vi "CV.vi"(2 "Run uninterrupted?":bool, 3 "Device Category:":string(combo)="Short Strip", 4 "Batch No.:":string, 5 "Wafer Serial No.:":string, 6 "Sensor Serial No.:":string) -> (0 "Done!":bool)   [LabVIEW 2013]
doc: "Performs CV measurements according to ATLAS ITk Quality Control Specifications."
uses:
  InstrControl/Switching/Switching.lvclass
  InstrControl/SupplyControl/SupplyControl.lvclass
  InstrControl/LCRControl/LCRControl.lvclass
  general_VIs/globals/QC_MeasurementSetup.vi
  general_VIs/globals/QC_RunInformation.vi
  InstrControl/InstrumentSetup.vi
  InstrControl/ArduinoControl/ArduinoControl.lvclass
  <vilib>/Analysis/NI_AALBase.lvlib
  InstrControl/InstrControl.lvclass
panel:
  out "Frequency [Hz]":i32=1000 format="%#.3p"
  out "Resistance":dbl[](array[numeric]) caption="Res [kOhm]"
  out "Initial volts [V]":dbl format="%.1f"
  out "Final volts [V]":dbl=-700.0 format="%.1f"
  out "step [V]":dbl=10.0 format="%.1f"
  out "step interval [s]":u32=5
  out "Volts":dbl[](array[numeric]) caption="Volts [V]"
  out "Capacitance":dbl[](array[numeric]) caption="Cap [pF]"
  out "Temp.":dbl[](array[numeric]) caption="Temp. [°C]" format="%#.2f"
  out "RH":dbl[](array[numeric]) caption="RH [%]" format="%#.2f"
  out "Cgraph":cluster{"Initial volts":dbl, dbl, dbl[]}(graph)
  in  "Scales":T1(ring)
  in  "Cscale":enum16{"1/C^2 [1/nF^2]", "nF", "pF"}(ring)
  out "positive ramp?":bool
  out "Tab Control":enum32{"CV Setup", "CV Scan"}(tab)
  in  "Frequency [Hz] Setup":i32=1000 caption="Frequency [Hz]" format="%#.3p"
  in  "LCR Meter":string(combo)="WayneKerr 6440B"
  in  "User:":string(combo)="Christoph"
  in  "CV Supply":string(combo)="Keithley 2410"
  in  "Configurations":bool
  in  "Set\ncurrent\nlimit?":bool
  in  "Current \nLimit \n[µA]":dbl=1000.0 min=0.0001 format="%.3f"
  in  "Manufacturer:":string(combo)="Hamamatsu"
  in  "Quit":bool
  in  "Continue":bool
  in  "Temperature":enum16{"Read Arduino", "Enter manually"}(ring)
  in  "abort":bool
  out "Device Category:":string
  out "Batch:":string
  out "Current Volts:":dbl format="%.2f"
  in  "quit (no save)":bool
  in  "Quit & Save":bool
  out "Bias On/Off:":bool
  out "STATUS 1":string
  out "Initiated:":string
  out "Sensor No.:":string
  out "No of steps":u32
  out "Current reading No.":u32
  out "Last reading at:":string
  # "University of\nCambridge"
  # "Strip Sensor QC: CV"
  # "CV Scan parameters:"
  # "Last 5 readings:"
  # "n-4"
  # "n-3"
  # "n-2"
  # "n-1"
  # "n"
  # "Vertical Scale:"
  # "DUT & Test Description"
  # "Hardware"
  # "DUT & Test Description:"
  # "Current status:"
  # "Rdg No:"
  # "out of"
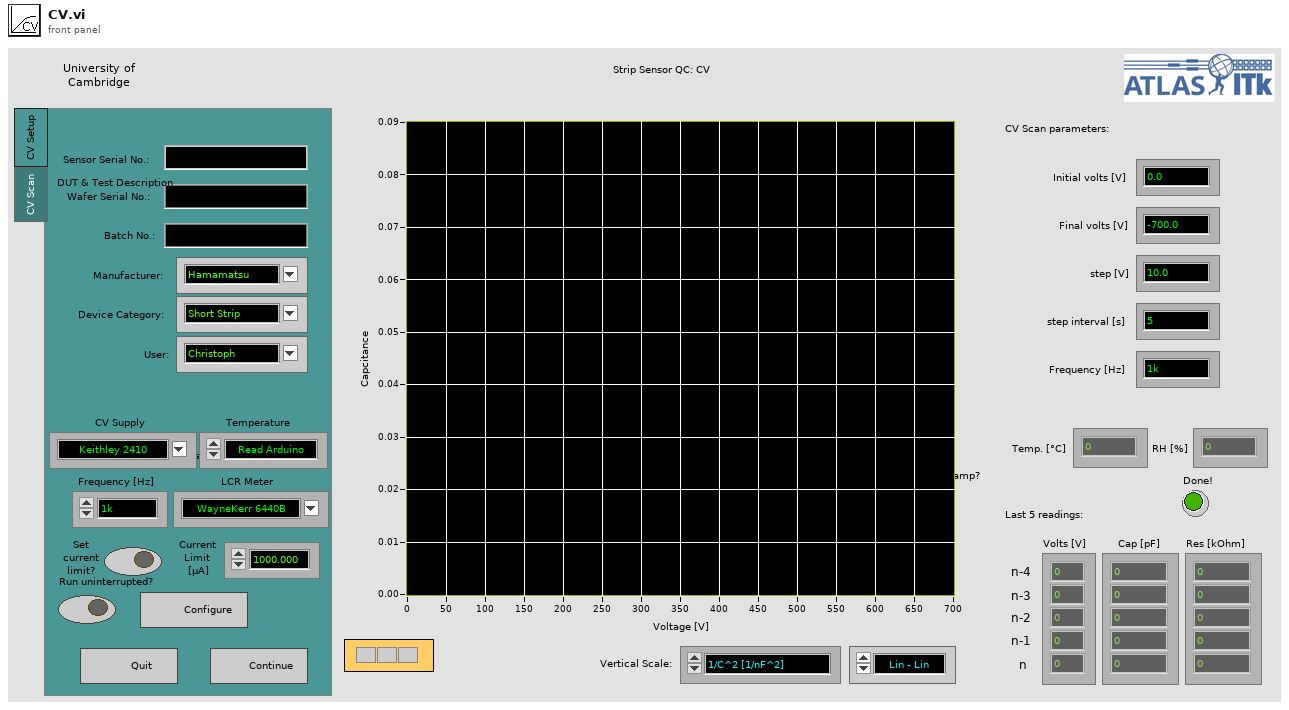
[diagram p1: front panel]
types:
  T1 = enum16{"Lin - Lin", "Log - Lin", "Lin - Log", "Log - log"}
  T2 = enum32{"IV", "CV", "Stability", "Striptest", "Cis", "Ris", "PTP"}
  T3 = enum16{"Reset", "Read Array", "Read Element", "Write Element", "Write Array", "Add Element", "Add Array"}
  T4 = enum16{"Reset", "Ground", "Striptest SMU", "Striptest LCR", "IV", "CV", "Interstrip Cap", "Interstrip Res"}
  T5 = cluster{"Sensor Serial No.:":string, "Wafer Serial No.:":string, "Batch:":string, "Manufacturer:":string, "Device Category:":string, "Database Serial No.:":string, "Initiated:":string, "Test":string, "Instruments used:":string, "Probeplan used:":string, "End of Run comment:":string, "User:":string}
  T6 = cluster{"Institute":string, "Manufacturers":string[], "Devices":string[], "Serialnumbers Lookup DB":string, "Data directory":string, "Backup & screenshot directory":string, "List of known users":string[]}
  T7 = cluster{"Supply":refnum<class "SupplyControl.lvclass">, "LCR":refnum<class "LCRControl.lvclass">, "Initial Voltage [V]":dbl, "Final Voltage [V]":dbl, "Step Size [V]":dbl, "Step Interval [s]":i32, "Number Of Steps":u32, "AC frequency [Hz]":i32, "RC Configuration":u16, "AC amplitude [V]":dbl, "Ramp down steps [V]":dbl, "Ramp down Interval [s]":i32, "Set Current Limit?":bool, "Current Limit [µA]":dbl, "Temperature Readout":enum16{"Read Arduino", "Enter manually"}, "Arduino":refnum<class "ArduinoControl.lvclass">, "Supply Name":string, "LCR Name":string, "V_depletion Limit [V]":dbl}
  T8 = cluster{"VISA address":refnum<visa-resource-name>, "T sensor":enum16{"SHT", "DS"}, "Arduino":refnum<class "ArduinoControl.lvclass">}
  T9 = cluster{"GPIB address":string, "Matrix address":string, "Mux1 address":string, "Mux2 address":string, "Matrix used?":bool, "Switching":refnum<class "Switching.lvclass">}
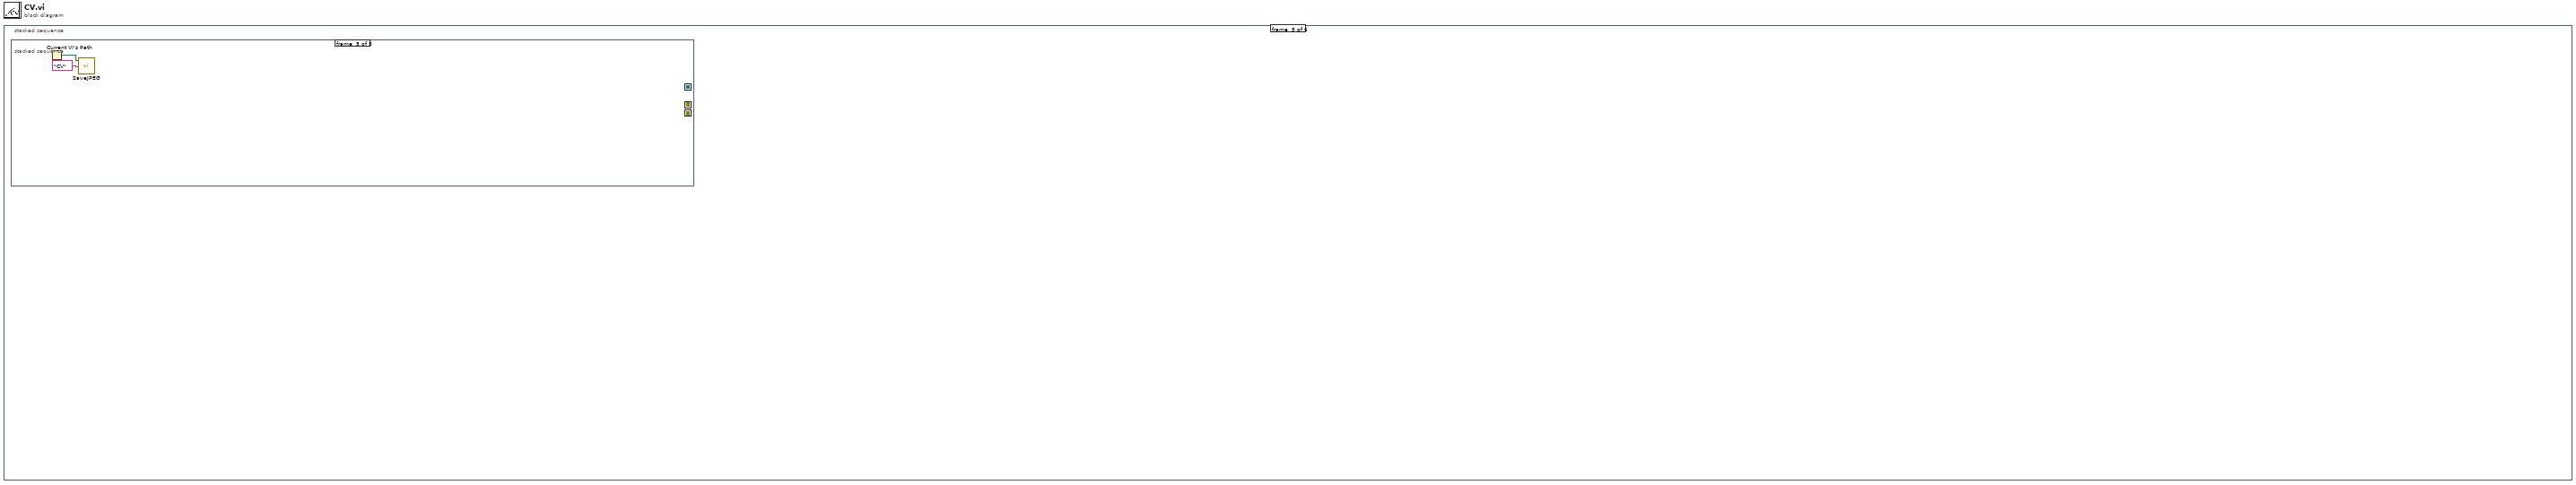
[diagram p0: block diagram]
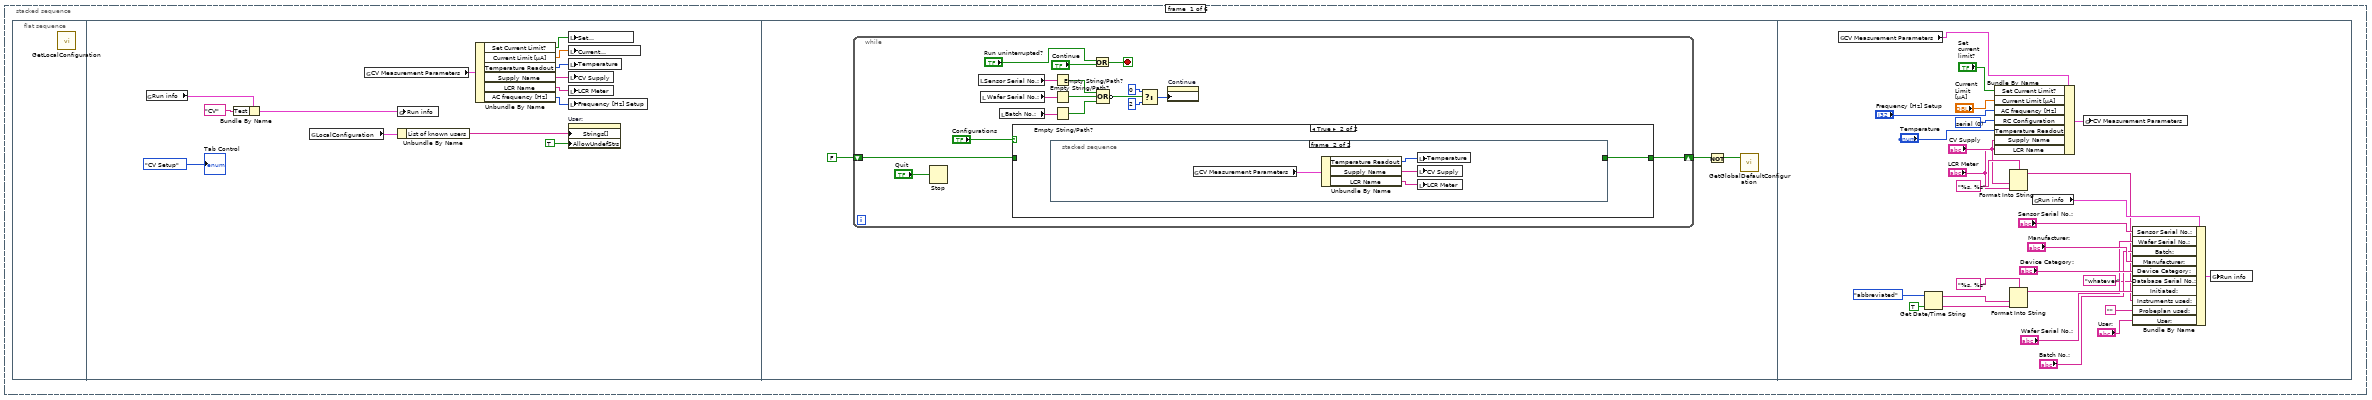
[diagram p2: hidden frame]
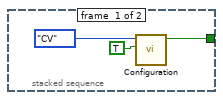
[diagram p4: hidden frame]
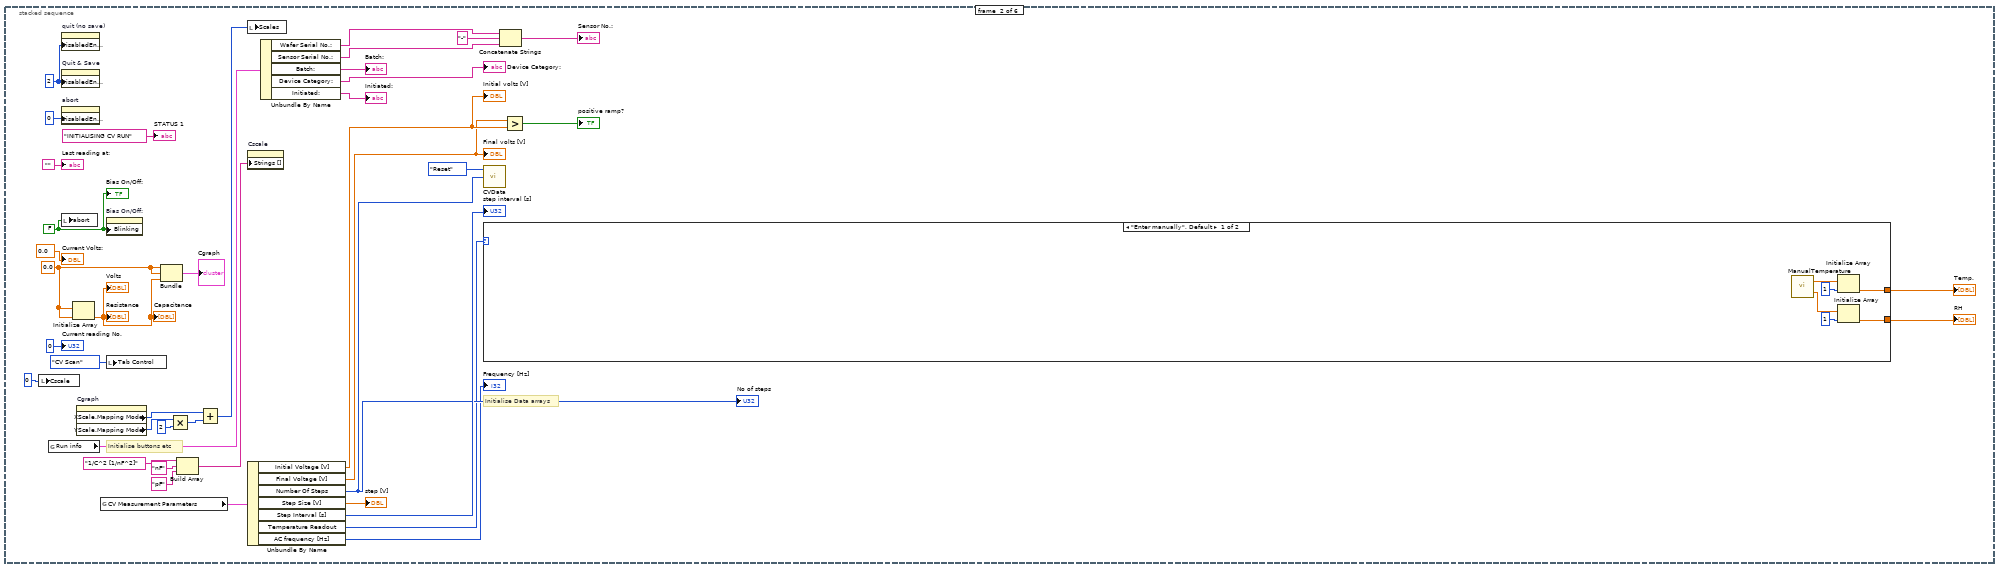
[diagram p5: hidden frame]
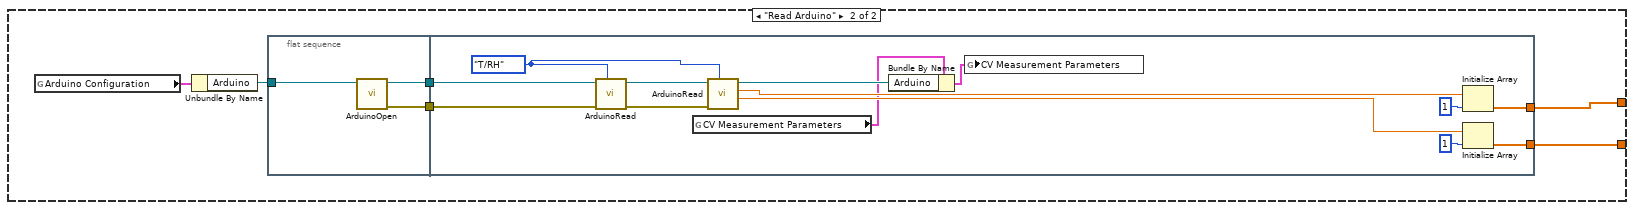
[diagram p6: hidden frame]
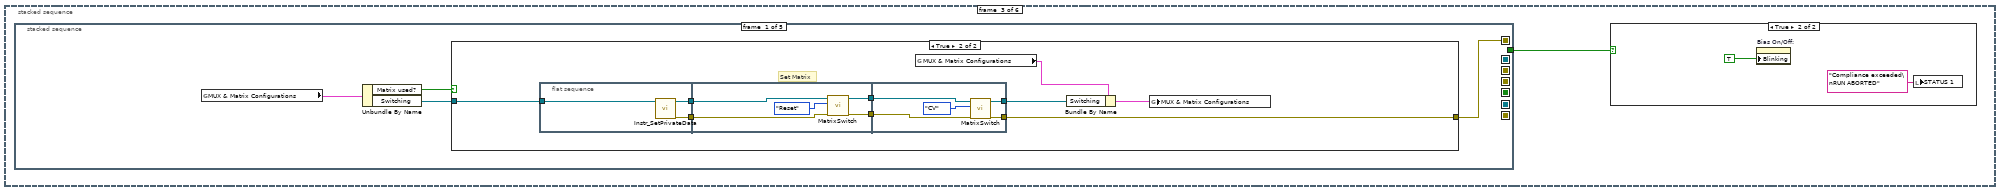
[diagram p7: hidden frame]
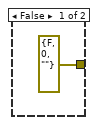
[diagram p8: hidden frame]
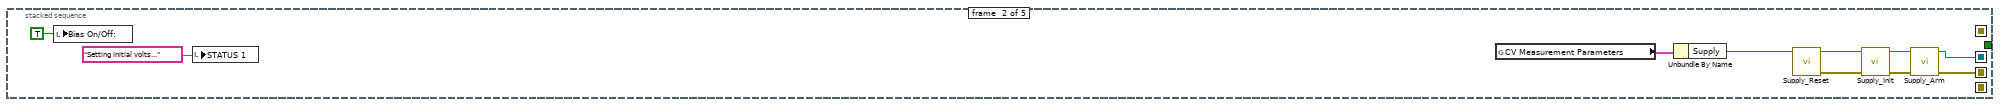
[diagram p9: hidden frame]
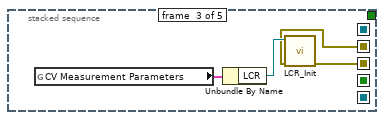
[diagram p10: hidden frame]
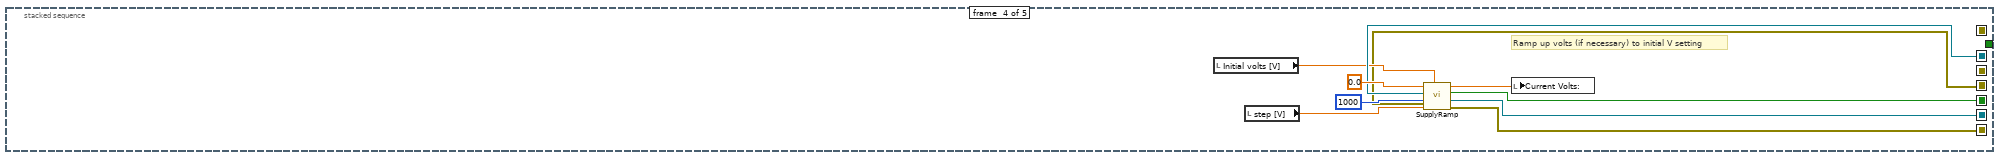
[diagram p11: hidden frame]
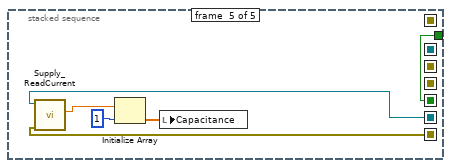
[diagram p12: hidden frame]
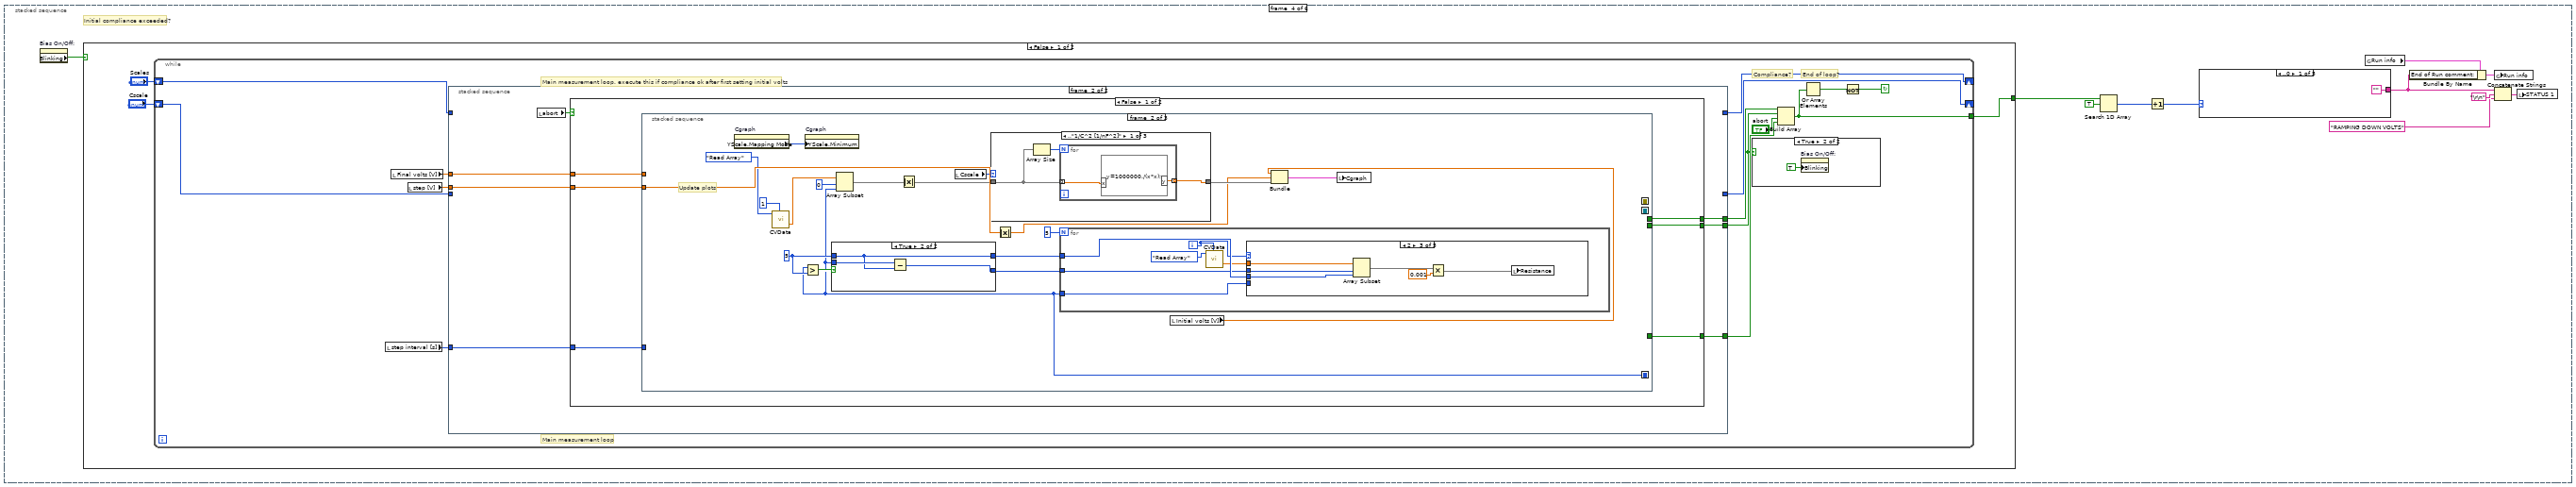
[diagram p14: hidden frame]
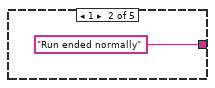
[diagram p15: hidden frame]
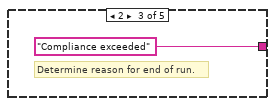
[diagram p16: hidden frame]
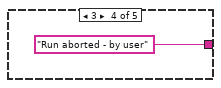
[diagram p17: hidden frame]
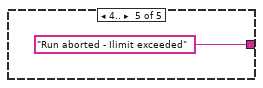
[diagram p18: hidden frame]
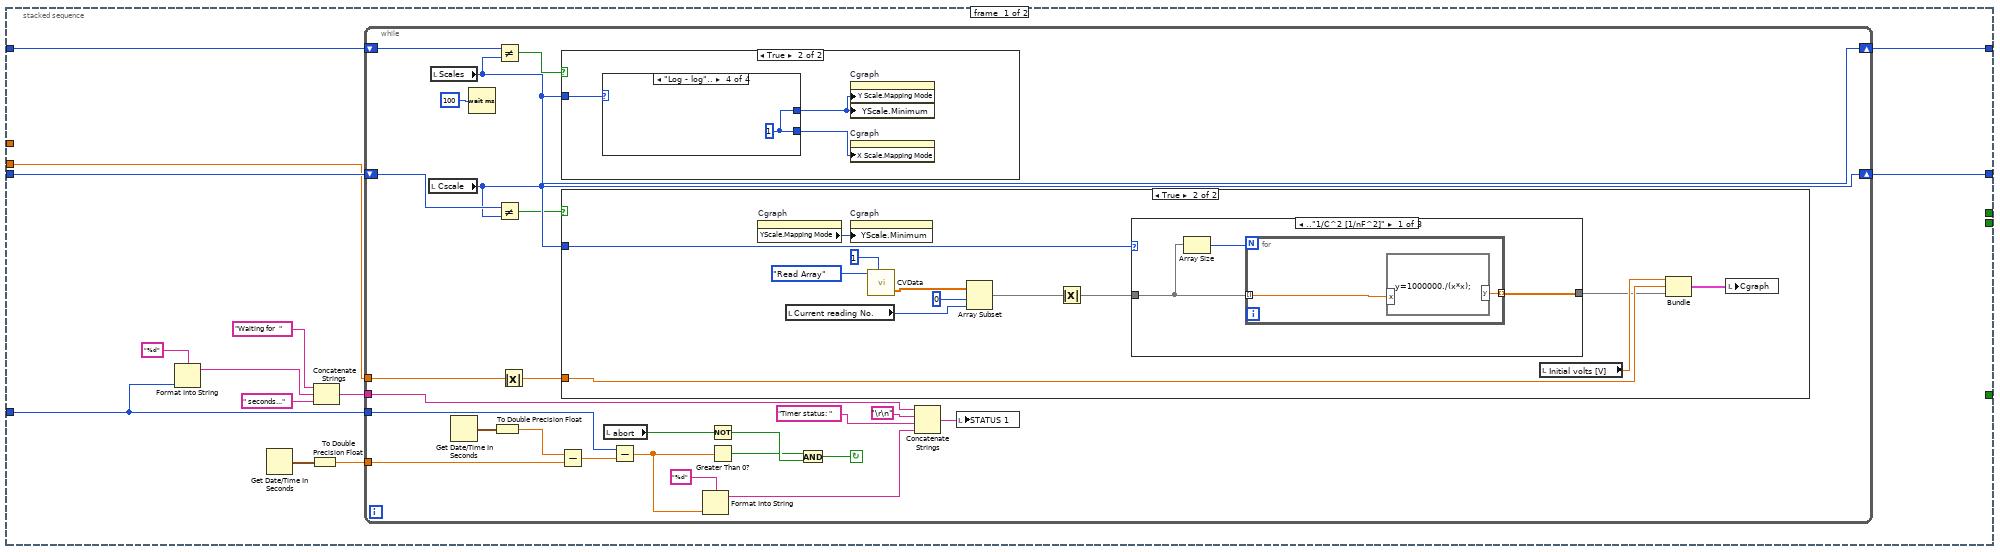
[diagram p19: hidden frame]
diagram:
  n1 = stacked-sequence {
    frame #0 {
      n2 = flat-sequence {
        frame #0 {
          n3 = call "GetLocalConfiguration.vi"() -> ()  [unwired: 3 in, 1 out]
        }
        frame #1 {
          n4 = global read "QC_RunInformation.vi" "Run info"() -> (w3:T5)
          n5 = Bundle By Name(cluster=w3, "Test"="CV") -> (w2:T5)
          n6 = global read "QC_RunInformation.vi" "LocalConfiguration"() -> (w9:T6)
          n7 = global read "QC_MeasurementSetup.vi" "CV Measurement Parameters"() -> (w12:T7)
          n8 = global write "QC_RunInformation.vi" "Run info"(w2) -> ()
          n9 = Unbundle By Name(w9) -> ("List of known users"=w8:string[])
          n10 = Unbundle By Name(w12) -> ("Set Current Limit?"=w11:bool, "Current Limit [µA]"=w10:dbl, "Temperature Readout"=w14:enum16{"Read Arduino", "Enter manually"}, "Supply Name"=w13:string, "LCR Name"=w5:string, "AC frequency [Hz]"=w4:i32)
          n11 = local write "Set\ncurrent\nlimit?"(w11) -> ()
          n12 = local write "Current \nLimit \n[µA]"(w10) -> ()
          n13 = local write "Temperature"(w14) -> ()
          n14 = local write "CV Supply"(w13) -> ()
          n15 = local write "LCR Meter"(w5) -> ()
          n16 = local write "Frequency [Hz] Setup"(w4) -> ()
          n17 = property on="User:" class="CmbBox"("Strings[]"=w8, "AllowUndefStrs"=TRUE) -> ()  [unwired: 2 in, 2 out]
          "Tab Control" <- enum32{"CV Setup", "CV Scan"}."CV Setup" ("Tab Control")
        }
        frame #2 {
          n18 = while {
            shift-right: [w22] -> w15
            shift-left: FALSE -> [w21]
            stop <- w18 stop-if-true
            n19 = Stop(stop? (T)="Quit") -> ()
            n20 = local read "Sensor Serial No.:"() -> (w33:string)
            n21 = local read "Wafer Serial No.:"() -> (w32:string)
            n22 = local read "Batch No.:"() -> (w24:string)
            n23 = case shown="True" "Configurations" {
              tunnel: [w35 w36] -> w22
              tunnel: w21 -> [w35 _]
              frame False {
              }
              frame True {
                n24 = stacked-sequence {
                  tunnel: [w37 _] -> w36
                  frame #0 {
                    n25 = call "Configuration.vi"("Open from\nscan VI"=TRUE, "Measurements"=T2."CV") -> ("configured?"=w37:bool)  [unwired: 9 in]
                  }
                  frame #1 {
                    n26 = global read "QC_MeasurementSetup.vi" "CV Measurement Parameters"() -> (w42:T7)
                    n27 = Unbundle By Name(w42) -> ("Temperature Readout"=w43:enum16{"Read Arduino", "Enter manually"}, "Supply Name"=w40:string, "LCR Name"=w41:string)
                    n28 = local write "Temperature"(w43) -> ()
                    n29 = local write "CV Supply"(w40) -> ()
                    n30 = local write "LCR Meter"(w41) -> ()
                  }
                }
              }
            }
            n31 = Empty String/Path?(string/path=w33) -> (empty?=w30:bool)
            n32 = Empty String/Path?(string/path=w32) -> (empty?=w31:bool)
            n33 = Empty String/Path?(string/path=w24) -> (empty?=w23:bool)
            n34 = Or(x="Run uninterrupted?", y="Continue") -> (x .or. y?=w18:bool)
            n35 = Compound Arithmetic op=OR(w30, w31, w23) -> (invert w29:bool)
            n36 = Select(t=0, s=w29, f=2) -> (s? t:f=w26:i32)
            n37 = property on="Continue" class="Bool"("DisabledEnum"=w26) -> ()  [unwired: 2 in, 2 out]
          }
          n38 = Not(x=w15) -> (.not. x?=w16:bool)
          n39 = call "GetGlobalDefaultConfiguration.vi"("Read defaults?"=w16) -> ()  [unwired: 2 in, 1 out]
        }
        frame #3 {
          w49 = u16 0 items=["serial", "parallel"] ("RC Configuration")
          n40 = global read "QC_MeasurementSetup.vi" "CV Measurement Parameters"() -> (w69:T7)
          n41 = Get Date/Time String(date format (0)=enum16{"short", "long", "abbreviated"}."abbreviated", want seconds? (F)=TRUE) -> (date string=w64:string, time string=w63:string)  [unwired: 1 in]
          n42 = Bundle By Name(cluster=w69, "Set Current Limit?"="Set\ncurrent\nlimit?", "Current Limit [µA]"="Current \nLimit \n[µA]", "AC frequency [Hz]"="Frequency [Hz] Setup", "RC Configuration"=w49, "Temperature Readout"="Temperature", "Supply Name"="CV Supply", "LCR Name"="LCR Meter") -> (w70:T7)
          n43 = Format Into String(format string="%s, %s", "CV Supply", "LCR Meter") -> (resulting string=w44:string)  [unwired: 2 in, 1 out]
          n44 = Format Into String(format string="%s, %s", w64, w63) -> (resulting string=w59:string)  [unwired: 2 in, 1 out]
          n45 = global read "QC_RunInformation.vi" "Run info"() -> (w61:T5)
          n46 = global write "QC_MeasurementSetup.vi" "CV Measurement Parameters"(w70) -> ()
          n47 = Bundle By Name(cluster=w61, "Sensor Serial No.:"="Sensor Serial No.:", "Wafer Serial No.:"="Wafer Serial No.:", "Batch:"="Batch No.:", "Manufacturer:"="Manufacturer:", "Device Category:"="Device Category:", "Database Serial No.:"="whatever", "Initiated:"=w59, "Instruments used:"=w44, "Probeplan used:"="", "User:"="User:") -> (w60:T5)
          n48 = global write "QC_RunInformation.vi" "Run info"(w60) -> ()
        }
      }
    }
    frame #1 {
      w93 = 2
      w100 = 0.0
      w92 = FALSE ("Visible")
      # "Initialise buttons etc"
      # "Initialise Data arrays"
      n49 = local write "Cscale"(u16 0 ("Scale")) -> ()
      n50 = global read "QC_RunInformation.vi" "Run info"() -> (w110:T5)
      n51 = property on="quit (no save)" class="Bool"("DisabledEnum"=w93) -> ()  [unwired: 2 in, 2 out]
      n52 = property on="Quit & Save" class="Bool"("DisabledEnum"=w93) -> ()  [unwired: 2 in, 2 out]
      n53 = property on="abort" class="Bool (strict)"("DisabledEnum"=0) -> ()  [unwired: 2 in, 2 out]
      n54 = local write "abort"(w92) -> ()
      n55 = Initialize Array(w100, w100) -> (w72:dbl[])
      "Volts" <- w72
      "Capacitance" <- w72
      "Resistance" <- w72
      n56 = property on="Cgraph" class="WFGraph (strict)"() -> ("XScale.Mapping Mode"=w85:u8, "YScale.Mapping Mode"=w84:u8)  [unwired: 2 in, 2 out]
      n57 = global read "QC_MeasurementSetup.vi" "CV Measurement Parameters"() -> (w81:T7)
      n58 = property on="Bias On/Off:" class="Bool (strict)"("Blinking"=w92) -> ()  [unwired: 2 in, 2 out]
      n59 = local write "Tab Control"(enum32{"CV Setup", "CV Scan"}."CV Scan" ("Tab Control")) -> ()
      n60 = Bundle(w100, w100, w72) -> (→"Cgraph":cluster{dbl, dbl, dbl[]})  [unwired: 1 in]
      n61 = Multiply(x=w84, y=2) -> (x*y=w87:i32)
      n62 = Build Array("1/C^2 [1/nF^2]", "nF", "pF") -> (w107:string[])
      n63 = Add(x=w85, y=w87) -> (x+y=w83:i32)
      n64 = local write "Scales"(w83) -> ()
      n65 = property on="Cscale" class="Enum (strict)"("Strings []"=w107) -> ()  [unwired: 2 in, 2 out]
      n66 = Unbundle By Name(w81) -> ("Initial Voltage [V]"=w91:dbl, "Final Voltage [V]"=w90:dbl, "Number Of Steps"=w101:u32, "Step Size [V]"=→"step [V]":dbl, "Step Interval [s]"=→"step interval [s]":i32, "Temperature Readout"=w94:enum16{"Read Arduino", "Enter manually"}, "AC frequency [Hz]"=→"Frequency [Hz]":i32)
      "No of steps" <- w101
      "Initial volts [V]" <- w91
      "Final volts [V]" <- w90
      n67 = Unbundle By Name(w110) -> ("Wafer Serial No.:"=w78:string, "Sensor Serial No.:"=w77:string, "Batch:"=→"Batch:":string, "Device Category:"=→"Device Category:":string, "Initiated:"=→"Initiated:":string)
      n68 = call "CVData.vi"("Action"=T3."Reset", "Array Size / Index"=w101) -> ()  [unwired: 3 in, 2 out]
      n69 = case shown="\"Enter manually\", Default" w94 {
        tunnel: [w116 w123] -> w97
        tunnel: [w113 w122] -> w82
        frame "Enter manually", Default {
          n70 = call "ManualTemperature.vi"() -> ("Humidity [%] out"=w112:dbl, "Temperature [°C] out"=w117:dbl)
          n71 = Initialize Array(w117, 1) -> (w116:dbl[])
          n72 = Initialize Array(w112, 1) -> (w113:dbl[])
        }
        frame "Read Arduino" {
          n73 = global read "InstrumentSetup.vi" "Arduino Configuration"() -> (w119:T8)
          n74 = Unbundle By Name(w119) -> ("Arduino"=w118:refnum<class "ArduinoControl.lvclass">)
          n75 = flat-sequence {
            tunnel: [w124] -> w121
            tunnel: [w126] -> w120
            tunnel: w118 -> [w125]
            tunnel: [w140] -> w123
            tunnel: [w137] -> w122
            tunnel: w121 -> [w129]
            tunnel: w120 -> [w130]
            frame #0 {
              n76 = call "ArduinoOpen.vi"("ArduinoControl in"=w125) -> ("error out"=w126:errorcluster, "ArduinoControl out"=w124:refnum<class "ArduinoControl.lvclass">)  [unwired: 9 in]
            }
            frame #1 {
              w131 = enum16{"T/RH", "Interlock", "Edgesense"}."T/RH" ("Arduino function")
              n77 = call "ArduinoRead.vi"("Arduino function"=w131, "error in (no error)"=w130, "ArduinoControl in"=w129) -> ("error out"=w127:errorcluster, "ArduinoControl out"=w128:refnum<class "ArduinoControl.lvclass">)  [unwired: 3 in, 4 out]
              n78 = global read "QC_MeasurementSetup.vi" "CV Measurement Parameters"() -> (w133:T7)
              n79 = call "ArduinoRead.vi"("Arduino function"=w131, "error in (no error)"=w127, "ArduinoControl in"=w128) -> ("rel. Humidity [%]"=w135:dbl, "Temperature [°C]"=w136:dbl, "ArduinoControl out"=w134:refnum<class "ArduinoControl.lvclass">)  [unwired: 3 in, 3 out]
              n80 = Bundle By Name(cluster=w133, "Arduino"=w134) -> (w132:T7)
              n81 = global write "QC_MeasurementSetup.vi" "CV Measurement Parameters"(w132) -> ()
              n82 = Initialize Array(w136, 1) -> (w140:dbl[])
              n83 = Initialize Array(w135, 1) -> (w137:dbl[])
            }
          }
        }
      }
      "Temp." <- w97
      "RH" <- w82
      n84 = Concatenate Strings(w78, "-", w77) -> (→"Sensor No.:":string)
      n85 = Greater?(x=w90, y=w91) -> (0:→"positive ramp?":bool)
      "STATUS 1" <- "INITIALISING CV RUN"
      "Bias On/Off:" <- w92
      "Last reading at:" <- ""
      "Current reading No." <- u32 0 ("Current reading No.")
      "Current Volts:" <- 0.0 ("Current Volts:")
    }
    frame #2 {
      n86 = stacked-sequence {
        seq-local: [_ w174 _ _ _] -> [_ _ _ w187 _]
        seq-local: [_ w173 _ _ _] -> [_ _ w180 _ _]
        seq-local: [_ _ _ w188 _] -> [_ _ _ _ w196]
        seq-local: [_ _ _ w186 _] -> [_ _ _ _ w197]
        seq-local: [_ _ _ w185 _] -> [_ _ _ _ w198]
        seq-local: [w142 _ _ _ _] -> [_ _ _ _ _]
        seq-local: [_ _ w179 _ _] -> [_ _ _ w183 _]
        tunnel: [_ _ _ _ w196] -> w141
        frame #0 {
          n87 = global read "InstrumentSetup.vi" "MUX & Matrix Configurations"() -> (w144:T9)
          n88 = Unbundle By Name(w144) -> ("Matrix used?"=w145:bool, "Switching"=w143:refnum<class "Switching.lvclass">)
          n89 = case shown="True" w145 {
            tunnel: w143 -> [_ w153]
            tunnel: [errorcluster {"status"=FALSE, "code"=0, "source"=""} ("error constant") w147] -> w142
            frame False {
            }
            frame True {
              # "Set Matrix"
              n90 = flat-sequence {
                tunnel: w153 -> [w158]
                tunnel: [w157] -> w152
                tunnel: [w156] -> w151
                tunnel: [w163] -> w155
                tunnel: [w162] -> w154
                tunnel: w152 -> [w161]
                tunnel: w151 -> [w160]
                tunnel: w155 -> [w168]
                tunnel: w154 -> [w167]
                tunnel: [w166] -> w148
                tunnel: [w165] -> w147
                frame #0 {
                  n91 = call-dynamic "Instr_SetPrivateData.vi"("Switching in"=w158) -> ("error out"=w156:errorcluster, "Switching out"=w157:refnum<class "Switching.lvclass">)  [unwired: 9 in]
                }
                frame #1 {
                  n92 = call "MatrixSwitch.vi"("error in (no error)"=w160, "Action"=T4."Reset", "Switching in"=w161) -> ("error out"=w163:errorcluster, "Switching out"=w162:refnum<class "Switching.lvclass">)  [unwired: 7 in]
                }
                frame #2 {
                  n93 = call "MatrixSwitch.vi"("error in (no error)"=w168, "Action"=T4."CV", "Switching in"=w167) -> ("error out"=w165:errorcluster, "Switching out"=w166:refnum<class "Switching.lvclass">)  [unwired: 7 in]
                }
              }
              n94 = global read "InstrumentSetup.vi" "MUX & Matrix Configurations"() -> (w149:T9)
              n95 = Bundle By Name(cluster=w149, "Switching"=w148) -> (w150:T9)
              n96 = global write "InstrumentSetup.vi" "MUX & Matrix Configurations"(w150) -> ()
            }
          }
        }
        frame #1 {
          n97 = local write "Bias On/Off:"(TRUE ("Compliance?")) -> ()
          n98 = local write "STATUS 1"("Setting initial volts..." ("STATUS 1")) -> ()
          n99 = global read "QC_MeasurementSetup.vi" "CV Measurement Parameters"() -> (w172:T7)
          n100 = Unbundle By Name(w172) -> ("Supply"=w169:refnum<class "SupplyControl.lvclass">)
          n101 = call-dynamic "Supply_Reset.vi"("SupplyControl in"=w169) -> ("error out"=w176:errorcluster, "SupplyControl out"=w178:refnum<class "SupplyControl.lvclass">)  [unwired: 9 in]
          n102 = call-dynamic "Supply_Init.vi"("error in (no error)"=w176, "SupplyControl in"=w178) -> ("error out"=w175:errorcluster, "SupplyControl out"=w177:refnum<class "SupplyControl.lvclass">)  [unwired: 8 in]
          n103 = call-dynamic "Supply_Arm.vi"("error in (no error)"=w175, "SupplyControl in"=w177) -> ("error out"=w173:errorcluster, "SupplyControl out"=w174:refnum<class "SupplyControl.lvclass">)  [unwired: 8 in]
        }
        frame #2 {
          n104 = global read "QC_MeasurementSetup.vi" "CV Measurement Parameters"() -> (w182:T7)
          n105 = Unbundle By Name(w182) -> ("LCR"=w181:refnum<class "LCRControl.lvclass">)
          n106 = call-dynamic "LCR_Init.vi"("error in (no error)"=w180, "LCRControl in"=w181) -> ("error out"=w179:errorcluster)  [unwired: 8 in, 1 out]
        }
        frame #3 {
          # "Ramp up volts (if necessary) to initial V setting"
          n107 = local read "Initial volts [V]"() -> (w184:dbl)
          n108 = local read "step [V]"() -> (w189:dbl)
          n109 = call "SupplyRamp.vi"("error in"=w183, "Requested Voltage"=w184, "Step Size"=w189, "Step Delay"=1000, "Supply IN"=w187, "Starting Voltage"=0.0) -> ("error out"=w186:errorcluster, "Supply OUT"=w185:refnum<class "SupplyControl.lvclass">, "Compliance exceeded"=w188:bool, "Current Voltage"=w192:dbl)  [unwired: 2 in]
          n110 = local write "Current Volts:"(w192) -> ()
        }
        frame #4 {
          n111 = call-dynamic "Supply_ReadCurrent.vi"("error in (no error)"=w197, "SupplyControl in"=w198) -> ("Current in nA"=w194:dbl)  [unwired: 7 in, 2 out]
          n112 = Initialize Array(w194, 1) -> (w193:dbl[])
          n113 = local write "Capacitance"(w193) -> ()
        }
      }
      n114 = case shown="True" w141 {
        frame False {
        }
        frame True {
          n115 = property on="Bias On/Off:" class="Bool (strict)"("Blinking"=TRUE) -> ()  [unwired: 2 in, 2 out]
          n116 = local write "STATUS 1"("Compliance exceeded\nRUN ABORTED") -> ()
        }
      }
    }
    frame #3 {
      # "Initial compliance exceeded?"
      n117 = property on="Bias On/Off:" class="Bool (strict)"() -> ("Blinking"=w211:bool)  [unwired: 2 in, 2 out]
      n118 = case shown="False" w211 {
        tunnel: [w219 w466] -> w210
        frame False {
          n119 = while {
            shift-left: "Cscale" -> [w229]
            shift-right: [w228] -> _
            shift-left: "Scales" -> [w230]
            shift-right: [w231] -> _
            tunnel: [w227] -> w219
            stop <- w232 continue-if-true
            # "Main measurement loop"
            # "End of loop?"
            # "Compliance?"
            # "Main measurement loop. execute this if compliance ok after first setting initial volts"
            n120 = local read "step interval [s]"() -> (w224:u32)
            n121 = local read "Final volts [V]"() -> (w225:dbl)
            n122 = local read "step [V]"() -> (w226:dbl)
            n123 = stacked-sequence {
              tunnel: [w246 _] -> w231
              tunnel: w226 -> [w243 w309]
              tunnel: [_ w308] -> w221
              tunnel: w225 -> [_ w307]
              tunnel: w224 -> [w234 w306]
              tunnel: [_ w305] -> w223
              tunnel: w230 -> [w245 _]
              tunnel: w229 -> [w244 _]
              tunnel: [w242 _] -> w228
              tunnel: [_ w303] -> w222
              frame #0 {
                n124 = Format Into String(format string="%d", w234) -> (resulting string=w239:string)  [unwired: 2 in, 1 out]
                n125 = Get Date/Time In Seconds() -> (seconds since 1Jan1904=w236:timestamp)
                n126 = To Double Precision Float(number=w236) -> (double precision float=w237:dbl)
                n127 = Concatenate Strings("Waiting for  ", w239, " seconds...") -> (w235:string)
                n128 = while {
                  tunnel: w243 -> [w255]
                  shift-left: w244 -> [w259]
                  shift-right: [w252] -> w242
                  shift-left: w245 -> [w260]
                  shift-right: [w261] -> w246
                  tunnel: w235 -> [w253]
                  tunnel: w234 -> [w265]
                  tunnel: w237 -> [w266]
                  stop <- w267 continue-if-true
                  n129 = local read "Cscale"() -> (w252:enum16{"1/C^2 [1/nF^2]", "nF", "pF"})
                  n130 = local read "Scales"() -> (w261:T1)
                  n131 = Get Date/Time In Seconds() -> (seconds since 1Jan1904=w251:timestamp)
                  n132 = Wait (ms)(milliseconds to wait=u32 100) -> ()  [unwired: 1 out]
                  n133 = To Double Precision Float(number=w251) -> (double precision float=w271:dbl)
                  n134 = Not Equal?(x=w260, y=w261) -> (x != y?=w262:bool)
                  n135 = Not Equal?(x=w259, y=w252) -> (x != y?=w250:bool)
                  n136 = Absolute Value(x=w255) -> (abs(x)=w254:dbl)
                  n137 = Subtract(x=w271, y=w266) -> (x-y=w248:dbl)
                  n138 = case shown="True" w262 {
                    tunnel: w261 -> [_ w296]
                    frame False {
                    }
                    frame True {
                      n139 = case shown="\"Log - log\".." w296 {
                        tunnel: [w297 1 0 w302] -> w295
                        tunnel: [w297 0 1 w302] -> w294
                        frame .."Lin - Lin" {
                          w297 = 0
                        }
                        frame "Log - Lin" {
                        }
                        frame "Lin - Log" {
                        }
                        frame "Log - log".. {
                          w302 = 1
                        }
                      }
                      n140 = property on="Cgraph" class="WFGraph (strict)"("Y Scale.Mapping Mode"=w294, "YScale.Minimum"=w294) -> ()  [unwired: 2 in, 2 out]
                      n141 = property on="Cgraph" class="WFGraph (strict)"("X Scale.Mapping Mode"=w295) -> ()  [unwired: 2 in, 2 out]
                    }
                  }
                  n142 = case shown="True" w250 {
                    tunnel: w254 -> [_ w283]
                    tunnel: w252 -> [_ w276]
                    frame False {
                    }
                    frame True {
                      n143 = property on="Cgraph" class="WFGraph (strict)"() -> ("YScale.Mapping Mode"=w278:u8)  [unwired: 2 in, 2 out]
                      n144 = local read "Current reading No."() -> (w281:u32)
                      n145 = property on="Cgraph" class="WFGraph (strict)"("YScale.Minimum"=w278) -> ()  [unwired: 2 in, 2 out]
                      n146 = call "CVData.vi"("Action"=T3."Read Array", "Array No."=u32 1 ("Action")) -> ("Array OUT"=w272:dbl[])  [unwired: 3 in, 1 out]
                      n147 = Array Subset(array=w272, index=0, length=w281) -> (w279:dbl[])
                      n148 = Absolute Value(x=w279) -> (abs(x)=w277:dbl[])
                      n149 = case shown="..\"1/C^2 [1/nF^2]\"" w276 {
                        tunnel: [w287 w290 w293] -> w275
                        tunnel: w277 -> [w285 w292 w293]
                        frame .."1/C^2 [1/nF^2]" {
                          n150 = Array Size(array=w285) -> (size(s)=w286:i32)
                          n151 = for {
                            N: w286 -> [_]
                            tunnel: w285 -> [w289] mode=indexing
                            tunnel: [w288] -> w287 mode=indexing
                            n152 = formula code="y=1000000./(x*x);"("x"=w289) -> ("y"=w288:dbl)
                          }
                        }
                        frame "nF" {
                          n153 = Divide(x=w292, y=1000.0) -> (x/y=w290:dbl[])
                        }
                        frame "pF".. {
                        }
                      }
                      n154 = local read "Initial volts [V]"() -> (w282:dbl)
                      n155 = Bundle("Initial volts [V]"=w282, w283, w275) -> (w280:cluster{"Initial volts [V]":dbl, dbl, dbl[]})  [unwired: 1 in]
                      n156 = local write "Cgraph"(w280) -> ()
                    }
                  }
                  n157 = local read "abort"() -> (w264:bool)
                  n158 = Subtract(x=w265, y=w248) -> (x-y=w247:dbl)
                  n159 = Format Into String(format string="%d", w247) -> (resulting string=w269:string)  [unwired: 2 in, 1 out]
                  n160 = Not(x=w264) -> (.not. x?=w270:bool)
                  n161 = Greater Than 0?(x=w247) -> (x > 0?=w249:bool)
                  n162 = And(x=w249, y=w270) -> (x .and. y?=w267:bool)
                  n163 = Concatenate Strings(w253, "\r\n", "Timer status: ", w269) -> (w263:string)
                  n164 = local write "STATUS 1"(w263) -> ()
                }
              }
              frame #1 {
                n165 = local read "abort"() -> (w304:bool)
                n166 = case shown="False" w304 {
                  tunnel: [w315 w463] -> w305
                  tunnel: w306 -> [w314 _]
                  tunnel: w307 -> [w313 _]
                  tunnel: [w311 w463] -> w308
                  tunnel: w309 -> [w312 _]
                  tunnel: [w310 w463] -> w303
                  frame False {
                    n167 = stacked-sequence {
                      seq-local: [w341 _ _] -> [_ w365 _]
                      seq-local: [w340 _ _] -> [_ _ w432]
                      seq-local: [w327 _ _] -> [_ _ w433]
                      tunnel: w312 -> [_ w377 w438]
                      tunnel: w313 -> [_ _ w429]
                      tunnel: [_ _ w436] -> w315
                      tunnel: [_ _ w435] -> w311
                      tunnel: w314 -> [_ _ _]
                      tunnel: [w343 _ _] -> w310
                      frame #0 {
                        w323 = T3."Write Element" ("Action")
                        # "SMU data"
                        n168 = Get Date/Time String(want seconds? (F)=TRUE) -> (time string=w342:string)  [unwired: 2 in, 1 out]
                        n169 = local write "Last reading at:"(w342) -> ()
                        n170 = local write "STATUS 1"("Reading LCR meter..." ("status")) -> ()
                        n171 = global read "QC_MeasurementSetup.vi" "CV Measurement Parameters"() -> (w339:T7)
                        n172 = Unbundle By Name(w339) -> ("Temperature Readout"=w317:enum16{"Read Arduino", "Enter manually"}, "Arduino"=w316:refnum<class "ArduinoControl.lvclass">, "LCR"=w333:refnum<class "LCRControl.lvclass">, "AC frequency [Hz]"=w318:i32, "Supply"=w334:refnum<class "SupplyControl.lvclass">, "Set Current Limit?"=w338:bool, "Current Limit [µA]"=w336:dbl)
                        n173 = case shown="\"Read Arduino\"" w317 {
                          tunnel: [w350 w353] -> w320
                          tunnel: [w347 w356] -> w325
                          tunnel: w316 -> [_ w355]
                          frame "Enter manually", Default {
                            n174 = local read "Temp."() -> (w352:dbl[])
                            n175 = local read "RH"() -> (w348:dbl[])
                            n176 = Index Array(array=w352, index=0) -> (element=w350:dbl)
                            n177 = Index Array(array=w348, index=0) -> (element=w347:dbl)
                          }
                          frame "Read Arduino" {
                            n178 = call "ArduinoRead.vi"("Arduino function"=enum16{"T/RH", "Interlock", "Edgesense"}."T/RH", "ArduinoControl in"=w355) -> ("rel. Humidity [%]"=w356:dbl, "Temperature [°C]"=w353:dbl)  [unwired: 4 in, 4 out]
                          }
                        }
                        n179 = Multiply(x=w336, y=1000.0) -> (x*y=w335:dbl)
                        n180 = local read "Current reading No."() -> (w322:u32)
                        n181 = call-dynamic "Supply_ReadCurrent.vi"("SupplyControl in"=w334) -> ("error out"=w328:errorcluster, "Current in nA"=w344:dbl, "SupplyControl out"=w340:refnum<class "SupplyControl.lvclass">)  [unwired: 8 in]
                        n182 = local read "Current Volts:"() -> (w326:dbl)
                        n183 = case shown="True" w338 {
                          tunnel: w344 -> [_ w361]
                          tunnel: w335 -> [_ w359]
                          tunnel: [FALSE w358] -> w343
                          frame False {
                          }
                          frame True {
                            n184 = Absolute Value(x=w361) -> (abs(x)=w360:dbl)
                            n185 = Greater?(x=w360, y=w359) -> (0:w358:bool)
                          }
                        }
                        n186 = call-dynamic "LCR_Readout.vi"("error in (no error)"=w328, "Frequency in Hz"=w318, "LCRControl in"=w333) -> ("error out"=w327:errorcluster, "Resistance in Ohm"=w321:dbl, "Capacitance in pF"=w319:dbl)  [unwired: 5 in, 1 out]
                        n187 = Increment(x=w322) -> (x+1=w341:u32)
                        n188 = local write "Current reading No."(w341) -> ()
                        n189 = call "CVData.vi"("Action"=w323, "Array No."=u32 1, "Array Size / Index"=w322, "Data IN"=w319) -> ()  [unwired: 1 in, 2 out]
                        n190 = call "CVData.vi"("Action"=w323, "Array No."=u32 2, "Array Size / Index"=w322, "Data IN"=w321) -> ()  [unwired: 1 in, 2 out]
                        n191 = call "CVData.vi"("Action"=w323, "Array No."=0, "Array Size / Index"=w322, "Data IN"=w326) -> ()  [unwired: 1 in, 2 out]
                        n192 = call "CVData.vi"("Action"=w323, "Array No."=u32 3, "Array Size / Index"=w322, "Data IN"=w320) -> ()  [unwired: 1 in, 2 out]
                        n193 = call "CVData.vi"("Action"=w323, "Array No."=u32 4, "Array Size / Index"=w322, "Data IN"=w325) -> ()  [unwired: 1 in, 2 out]
                      }
                      frame #1 {
                        w374 = u32 5 ("y")
                        # "Update plots"
                        n194 = property on="Cgraph" class="WFGraph (strict)"() -> ("YScale.Mapping Mode"=w366:u8)  [unwired: 2 in, 2 out]
                        n195 = call "CVData.vi"("Action"=T3."Read Array", "Array No."=1) -> ("Array OUT"=w363:dbl[])  [unwired: 3 in, 1 out]
                        n196 = Greater?(x=w365, y=w374) -> (0:w373:bool)
                        n197 = property on="Cgraph" class="WFGraph (strict)"("YScale.Minimum"=w366) -> ()  [unwired: 2 in, 2 out]
                        n198 = case shown="True" w373 {
                          tunnel: w365 -> [w382 w385]
                          tunnel: w374 -> [_ w384]
                          tunnel: [w382 w384] -> w372
                          tunnel: [0 w383] -> w370
                          frame False {
                          }
                          frame True {
                            n199 = Subtract(x=w385, y=w384) -> (x-y=w383:u32)
                          }
                        }
                        n200 = Array Subset(array=w363, index=0, length=w365) -> (w369:dbl[])
                        n201 = Absolute Value(x=w369) -> (abs(x)=w368:dbl[])
                        n202 = local read "Cscale"() -> (w375:enum16{"1/C^2 [1/nF^2]", "nF", "pF"})
                        n203 = case shown="..\"1/C^2 [1/nF^2]\"" w375 {
                          tunnel: [w418 w421 w424] -> w380
                          tunnel: w368 -> [w416 w423 w424]
                          frame .."1/C^2 [1/nF^2]" {
                            n204 = Array Size(array=w416) -> (size(s)=w417:i32)
                            n205 = for {
                              N: w417 -> [_]
                              tunnel: w416 -> [w420] mode=indexing
                              tunnel: [w419] -> w418 mode=indexing
                              n206 = formula code="y=1000000./(x*x);"("x"=w420) -> ("y"=w419:dbl)
                            }
                          }
                          frame "nF" {
                            n207 = Divide(x=w423, y=1000.0) -> (x/y=w421:dbl[])
                          }
                          frame "pF".. {
                          }
                        }
                        n208 = Absolute Value(x=w377) -> (abs(x)=w376:dbl)
                        n209 = for {
                          N: 5 -> [_]
                          tunnel: w372 -> [w391]
                          tunnel: w370 -> [w390]
                          tunnel: w365 -> [w389]
                          i -> [w387]
                          n210 = call "CVData.vi"("Action"=T3."Read Array", "Array No."=w387) -> ("Array OUT"=w386:dbl[])  [unwired: 3 in, 1 out]
                          n211 = case shown="2" w387 {
                            tunnel: w391 -> [w394 w398 w403 _ _]
                            tunnel: w390 -> [w395 w399 w404 _ _]
                            tunnel: w386 -> [w393 w397 w405 w409 w414]
                            tunnel: w389 -> [_ _ _ w407 w412]
                            frame ..0 {
                              n212 = Array Subset(array=w393, index=w395, length=w394) -> (w392:dbl[])
                              n213 = local write "Volts"(w392) -> ()
                            }
                            frame 1 {
                              n214 = Array Subset(array=w397, index=w399, length=w398) -> (w396:dbl[])
                              n215 = local write "Capacitance"(w396) -> ()
                            }
                            frame 2 {
                              n216 = Array Subset(array=w405, index=w404, length=w403) -> (w402:dbl[])
                              n217 = Multiply(x=w402, y=0.001) -> (x*y=w401:dbl[])
                              n218 = local write "Resistance"(w401) -> ()
                            }
                            frame 3 {
                              n219 = Decrement(x=w407) -> (x-1=w406:u32)
                              n220 = Array Subset(array=w409, index=w406, length=1) -> (w408:dbl[])
                              n221 = local write "Temp."(w408) -> ()
                            }
                            frame 4.. {
                              n222 = Decrement(x=w412) -> (x-1=w411:u32)
                              n223 = Array Subset(array=w414, index=w411, length=1) -> (w413:dbl[])
                              n224 = local write "RH"(w413) -> ()
                            }
                          }
                        }
                        n225 = local read "Initial volts [V]"() -> (w378:dbl)
                        n226 = Bundle("Initial volts [V]"=w378, w376, w380) -> (w367:cluster{"Initial volts [V]":dbl, dbl, dbl[]})  [unwired: 1 in]
                        n227 = local write "Cgraph"(w367) -> ()
                      }
                      frame #2 {
                        # "Increment volts and check for end of loop"
                        n228 = local read "positive ramp?"() -> (w434:bool)
                        n229 = local read "Current Volts:"() -> (w430:dbl)
                        n230 = Quotient & Remainder(x=w430, y=w429) -> (x-y*floor(x/y)=w431:dbl, floor(x/y)=w428:dbl)
                        n231 = case shown="True" w434 {
                          tunnel: w429 -> [w441 w445]
                          tunnel: w438 -> [w442 w448]
                          tunnel: [w440 w447] -> w425
                          tunnel: [w439 w444] -> w437
                          tunnel: w430 -> [w443 w446]
                          frame False {
                            n232 = Subtract(x=w443, y=w442) -> (x-y=w439:dbl)
                            n233 = Greater Or Equal?(x=w439, y=w441) -> (x >= y?=w440:bool)
                          }
                          frame True {
                            n234 = Add(x=w446, y=w448) -> (x+y=w444:dbl)
                            n235 = Less Or Equal?(x=w444, y=w445) -> (x <= y?=w447:bool)
                          }
                        }
                        n236 = Not Equal To 0?(x=w431) -> (x != 0?=w426:bool)
                        n237 = Equal To 0?(x=w428) -> (x = 0?=w427:bool)
                        n238 = Or(x=w426, y=w427) -> ()  [unwired: 1 out]
                        n239 = case shown="True" w425 {
                          tunnel: w437 -> [_ w459]
                          tunnel: [TRUE FALSE] -> w436
                          tunnel: [FALSE w460] -> w435
                          tunnel: w430 -> [_ w457]
                          tunnel: w433 -> [_ w456]
                          tunnel: w432 -> [_ w455]
                          frame False {
                          }
                          frame True {
                            n240 = local read "step [V]"() -> (w453:dbl)
                            n241 = local write "STATUS 1"("Incrementing volts.") -> ()
                            n242 = call "SupplyRamp.vi"("error in"=w456, "Requested Voltage"=w459, "Step Size"=w453, "Step Delay"=100, "Supply IN"=w455, "Starting Voltage"=w457) -> ("error out"=w451:errorcluster, "Compliance exceeded"=w460:bool, "Current Voltage"=w454:dbl)  [unwired: 2 in, 1 out]
                            n243 = property on="Bias On/Off:" class="Bool (strict)"("Blinking"=w460) -> ()  [unwired: 2 in, 2 out]
                            n244 = case shown="No Error" w451 {
                              tunnel: w454 -> [w462 _]
                              frame No Error {
                                n245 = local write "Current Volts:"(w462) -> ()
                              }
                              frame Error {
                              }
                            }
                          }
                        }
                      }
                    }
                  }
                  frame True {
                    w463 = FALSE
                  }
                }
              }
            }
            n246 = case shown="True" w221 {
              frame False {
              }
              frame True {
                n247 = property on="Bias On/Off:" class="Bool (strict)"("Blinking"=TRUE) -> ()  [unwired: 2 in, 2 out]
              }
            }
            n248 = Build Array(w223, w221, "abort", w222) -> (w227:bool[])
            n249 = Or Array Elements(Boolean array=w227) -> (logical OR=w233:bool)
            n250 = Not(x=w233) -> (.not. x?=w232:bool)
          }
        }
        frame True {
          w465 = FALSE
          # "compliance was exceeded when first voltage applied."
          # "Flag compliance as reason for end of run"
          n251 = local write "STATUS 1"("Run aborted - compliance exceeded.") -> ()
          n252 = Build Array(w465, TRUE, w465, w465) -> (w466:bool[])
        }
      }
      n253 = Search 1D Array(1D array=w210, element=TRUE) -> (index of element=w208:i32)  [unwired: 1 in]
      n254 = Increment(x=w208) -> (x+1=w207:i32)
      n255 = case shown="..0" w207 {
        tunnel: ["" "Run ended normally" "Compliance exceeded" "Run aborted - by user" "Run aborted - Ilimit exceeded"] -> w202
        frame ..0 {
        }
        frame 1 {
        }
        frame 2 {
          # "Determine reason for end of run."
        }
        frame 3 {
        }
        frame 4.. {
        }
      }
      n256 = global read "QC_RunInformation.vi" "Run info"() -> (w206:T5)
      n257 = Bundle By Name(cluster=w206, "End of Run comment:"=w202) -> (w201:T5)
      n258 = global write "QC_RunInformation.vi" "Run info"(w201) -> ()
      n259 = Concatenate Strings(w202, "\r\n", "RAMPING DOWN VOLTS") -> (w205:string)
      n260 = local write "STATUS 1"(w205) -> ()
    }
    frame #4 {
      n261 = stacked-sequence {
        seq-local: [w471 _ _ _ _] -> [_ w482 _ _ _]
        seq-local: [w470 _ _ _ _] -> [_ w481 _ _ _]
        seq-local: [_ w480 _ _ _] -> [_ _ w483 _ _]
        frame #0 {
          # "Ramp down volts now"
          n262 = global read "QC_MeasurementSetup.vi" "CV Measurement Parameters"() -> (w474:T7)
          n263 = Unbundle By Name(w474) -> ("Supply"=w469:refnum<class "SupplyControl.lvclass">, "Ramp down steps [V]"=w473:dbl, "Ramp down Interval [s]"=w472:i32)
          n264 = Multiply(x=w472, y=1000) -> (x*y=w476:i32)
          n265 = local read "Current Volts:"() -> (w479:dbl)
          n266 = call "SupplyRamp.vi"("Requested Voltage"=0.0, "Step Size"=w473, "Step Delay"=w476, "Supply IN"=w469, "Starting Voltage"=w479) -> ("error out"=w471:errorcluster, "Supply OUT"=w470:refnum<class "SupplyControl.lvclass">, "Current Voltage"=w477:dbl)  [unwired: 3 in, 1 out]
          n267 = local write "Current Volts:"(w477) -> ()
        }
        frame #1 {
          # "Tie up loose ends. Set volts to zero and switch to standby"
          n268 = call-dynamic "Supply_Stby.vi"("error in (no error)"=w482, "SupplyControl in"=w481) -> ("error out"=w480:errorcluster)  [unwired: 8 in, 1 out]
        }
        frame #2 {
          n269 = global read "InstrumentSetup.vi" "MUX & Matrix Configurations"() -> (w485:T9)
          n270 = Unbundle By Name(w485) -> ("Matrix used?"=w486:bool, "Switching"=w484:refnum<class "Switching.lvclass">)
          n271 = case shown="True" w486 {
            tunnel: w484 -> [_ w489]
            tunnel: w483 -> [_ w488]
            frame False {
            }
            frame True {
              n272 = call "MatrixSwitch.vi"("error in (no error)"=w488, "Action"=T4."Reset", "Switching in"=w489) -> ()  [unwired: 7 in, 2 out]
            }
          }
        }
        frame #3 {
          w494 = 0
          n273 = local write "Bias On/Off:"(FALSE ("Visible")) -> ()
          n274 = local write "Current Volts:"(0.0 ("Current Volts:")) -> ()
          n275 = property on="Quit & Save" class="Bool"("DisabledEnum"=w494) -> ()  [unwired: 2 in, 2 out]
          n276 = property on="quit (no save)" class="Bool"("DisabledEnum"=w494) -> ()  [unwired: 2 in, 2 out]
          n277 = property on="abort" class="Bool (strict)"("DisabledEnum"=2) -> ()  [unwired: 2 in, 2 out]
          n278 = local write "STATUS 1"("Run finished. \nSave data?" ("STATUS 1")) -> ()
        }
        frame #4 {
          n279 = Current VI's Path() -> (path=w496:path)
          n280 = call "SaveJPEG.vi"("Test"="CV", "File Path Control"=w496) -> ()  [unwired: 1 in, 2 out]
        }
      }
    }
    frame #5 {
      # "Loop and await decision on whether to save or junk data"
      n281 = local read "Cscale"() -> (w506:enum16{"1/C^2 [1/nF^2]", "nF", "pF"})
      n282 = local read "Scales"() -> (w507:T1)
      n283 = while {
        shift-left: w506 -> [w555]
        shift-right: [w554] -> _
        shift-left: w507 -> [w557]
        shift-right: [w556] -> _
        tunnel: ["Quit & Save"] -> w509
        tunnel: ["quit (no save)"] -> w508
        stop <- w552 continue-if-true
        n284 = local read "Cscale"() -> (w554:enum16{"1/C^2 [1/nF^2]", "nF", "pF"})
        n285 = local read "Scales"() -> (w556:T1)
        n286 = Not Equal?(x=w557, y=w556) -> (x != y?=w550:bool)
        n287 = Not Equal?(x=w555, y=w554) -> (x != y?=w549:bool)
        n288 = case shown="True" w550 {
          tunnel: w556 -> [_ w584]
          frame False {
          }
          frame True {
            n289 = case shown="..\"Lin - Lin\"" w584 {
              tunnel: [w585 1 0 w590] -> w583
              tunnel: [w585 0 1 w590] -> w582
              frame .."Lin - Lin" {
                w585 = 0
              }
              frame "Log - Lin" {
              }
              frame "Lin - Log" {
              }
              frame "Log - log".. {
                w590 = 1
              }
            }
            n290 = property on="Cgraph" class="WFGraph (strict)"("X Scale.Mapping Mode"=w583) -> ()  [unwired: 2 in, 2 out]
            n291 = property on="Cgraph" class="WFGraph (strict)"("Y Scale.Mapping Mode"=w582, "YScale.Minimum"=w582) -> ()  [unwired: 2 in, 2 out]
          }
        }
        n292 = case shown="True" w549 {
          tunnel: w554 -> [_ w562]
          frame False {
          }
          frame True {
            n293 = property on="Cgraph" class="WFGraph (strict)"() -> ("YScale.Mapping Mode"=w565:u8)  [unwired: 2 in, 2 out]
            n294 = property on="Cgraph" class="WFGraph (strict)"("YScale.Minimum"=w565) -> ()  [unwired: 2 in, 2 out]
            n295 = global read "QC_MeasurementSetup.vi" "CV Measurement Parameters"() -> (w564:T7)
            n296 = Unbundle By Name(w564) -> ("Initial Voltage [V]"=w567:dbl, "Step Size [V]"=w569:dbl, "Number Of Steps"=w566:u32)
            n297 = call "CVData.vi"("Action"=T3."Read Array", "Array No."=u32 1 ("Action")) -> ("Array OUT"=w558:dbl[])  [unwired: 3 in, 1 out]
            n298 = Array Subset(array=w558, index=0, length=w566) -> (w570:dbl[])
            n299 = Absolute Value(x=w570) -> (abs(x)=w563:dbl[])
            n300 = case shown="..\"1/C^2 [1/nF^2]\"" w562 {
              tunnel: [w575 w578 w581] -> w561
              tunnel: w563 -> [w573 w580 w581]
              frame .."1/C^2 [1/nF^2]" {
                n301 = Array Size(array=w573) -> (size(s)=w574:i32)
                n302 = for {
                  N: w574 -> [_]
                  tunnel: w573 -> [w577] mode=indexing
                  tunnel: [w576] -> w575 mode=indexing
                  n303 = formula code="y=1000000./(x*x);"("x"=w577) -> ("y"=w576:dbl)
                }
              }
              frame "nF" {
                n304 = Divide(x=w580, y=1000.0) -> (x/y=w578:dbl[])
              }
              frame "pF".. {
              }
            }
            n305 = Absolute Value(x=w569) -> (abs(x)=w568:dbl)
            n306 = Bundle("Initial Voltage [V]"=w567, w568, w561) -> (w571:cluster{"Initial Voltage [V]":dbl, dbl, dbl[]})  [unwired: 1 in]
            n307 = local write "Cgraph"(w571) -> ()
          }
        }
        n308 = Not Or(1:"quit (no save)", 2:"Quit & Save") -> (0:w552:bool)
      }
      n309 = global read "QC_MeasurementSetup.vi" "CV Measurement Parameters"() -> (w505:T7)
      n310 = Unbundle By Name(w505) -> ("Temperature Readout"=w504:enum16{"Read Arduino", "Enter manually"}, "Arduino"=w498:refnum<class "ArduinoControl.lvclass">)
      n311 = case shown="\"Read Arduino\"" w504 {
        tunnel: w498 -> [_ w548]
        frame "Enter manually", Default {
        }
        frame "Read Arduino" {
          n312 = call "ArduinoClose.vi"("ArduinoControl in"=w548) -> ()  [unwired: 9 in, 2 out]
        }
      }
      n313 = case shown="True" w508 {
        tunnel: [FALSE w592] -> w510
        frame False {
        }
        frame True {
          n314 = Two Button Dialog(message="Are you sure you don't want to save the data?", 1:"Quit" ("F button name (\"Cancel\")"), 2:"Save data" ("T button name (\"OK\")")) -> (T button?=w592:bool)
        }
      }
      n315 = Or(x=w509, y=w510) -> (x .or. y?=w503:bool)
      n316 = flat-sequence {
        tunnel: w503 -> [w511]
        tunnel: [w511] -> w499
        tunnel: [TRUE] -> w497
        frame #0 {
          n317 = global read "QC_MeasurementSetup.vi" "CV Measurement Parameters"() -> (w521:T7)
          n318 = Unbundle By Name(w521) -> ("V_depletion Limit [V]"=w513:dbl, "Number Of Steps"=w516:u32)
          n319 = Absolute Value(x=w513) -> (abs(x)=w512:dbl)
          n320 = case shown="True" w511 {
            tunnel: ["" w547] -> w522
            tunnel: [_ w530] -> w520
            tunnel: w516 -> [_ w527]
            frame False {
            }
            frame True {
              w528 = T3."Read Array" ("Action")
              n321 = local write "STATUS 1"("Saving Data ...") -> ()
              n322 = call "CVData.vi"("Action"=w528, "Array No."=u32 4 ("Action")) -> ("Array OUT"=w543:dbl[])  [unwired: 3 in, 1 out]
              n323 = call "CVData.vi"("Action"=w528, "Array No."=u32 3 ("Action")) -> ("Array OUT"=w542:dbl[])  [unwired: 3 in, 1 out]
              n324 = call "CVData.vi"("Action"=w528, "Array No."=u32 2 ("Action")) -> ("Array OUT"=w525:dbl[])  [unwired: 3 in, 1 out]
              n325 = call <vilib>:"Std Deviation and Variance.vi"("X"=w543) -> ("mean"=w531:dbl)  [unwired: 1 in, 2 out]
              n326 = call <vilib>:"Std Deviation and Variance.vi"("X"=w542) -> ("mean"=w532:dbl)  [unwired: 1 in, 2 out]
              n327 = Multiply(x=w525, y=0.001) -> (x*y=w524:dbl[])
              n328 = call "CVData.vi"("Action"=w528, "Array No."=u32 0 ("Action")) -> ("Array OUT"=w537:dbl[])  [unwired: 3 in, 1 out]
              n329 = call "CVData.vi"("Action"=w528, "Array No."=u32 1 ("Action")) -> ("Array OUT"=w536:dbl[])  [unwired: 3 in, 1 out]
              n330 = Build Array(w537, w536, w524) -> (w535:dbl[][])
              n331 = Transpose 2D Array(2D array=w535) -> (transposed array=w534:dbl[][])
              n332 = call "SaveDataFile.vi"("Arrays format"="%010.2f", "Humidity"=w531, "Array Titles"="Voltage[V] Capacitance[pF] Resistance[kOhm]", "Temperature"=w532, "Actual array lengths"=w527, "no. of arrays"=3, "Data Array"=w534) -> ("Error Out"=w530:errorcluster, "Path + Filename OUT"=w547:string)  [unwired: 1 in, 2 out]
            }
          }
          n333 = call "ScanFeedback.vi"("measurement type"=T2."CV") -> ("V depletion"=w515:dbl)  [unwired: 3 in, 5 out]
          n334 = Absolute Value(x=w515) -> (abs(x)=w514:dbl)
          n335 = Less Or Equal?(x=w514, y=w512) -> (x <= y?=w517:bool)
          n336 = call "WriteLogFile.vi"("Data File"=w522, "Error In"=w520, "DUT passed?"=w517, "Value TechSpec criteria"=w515, "Files saved?"=w511) -> ()  [unwired: 6 in, 1 out]
        }
      }
      n337 = Select(t="Run finished.\nData saved." ("STATUS 1"), s=w499, f="Run finished.\nData not saved." ("STATUS 1")) -> (s? t:f=w502:string)
      n338 = local write "STATUS 1"(w502) -> ()
      "Done!" <- w497
    }
  }
